vi "Handle TS Panel Results.vi"(6 "Method":T1, 8 "error in":errorcluster, 11 "HTS Test Stand in":refnum<class "HTS Test Stand.lvclass">) -> (0 "error out":errorcluster, 3 "HTS Test Stand out":refnum<class "HTS Test Stand.lvclass">)   [LabVIEW 2019, in "Test Stands.lvlib" / "HTS Test Stand.lvclass"]
uses:
  HTS Test Stand.lvclass
  Results/Results Method.ctl
  Results/Results.lvlib
  Generic Test Stand/Generic Test Stand.lvclass
  C:/Users/wg/Documents/LV_Projects/test-stand/App/Generic Test Stand/Generic Test Stand.lvclass
  Results/HTS Results/HTS Results.lvclass
  Generic Test Stand/TS Panel Method.ctl
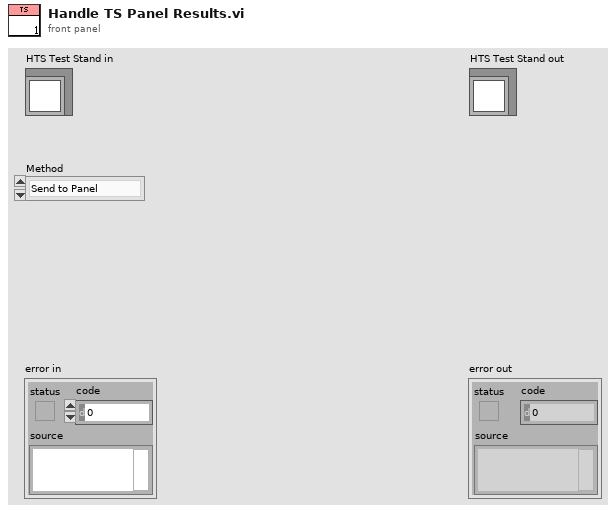
[diagram p1: front panel]
types:
  T1 = typedef "Generic Test Stand.lvclass/TS Panel Method.ctl" = enum16{"Send to Panel", "Receive from Panel"}
  T2 = typedef "Results.lvlib/Results Method.ctl" = enum16{"Get", "Set"}
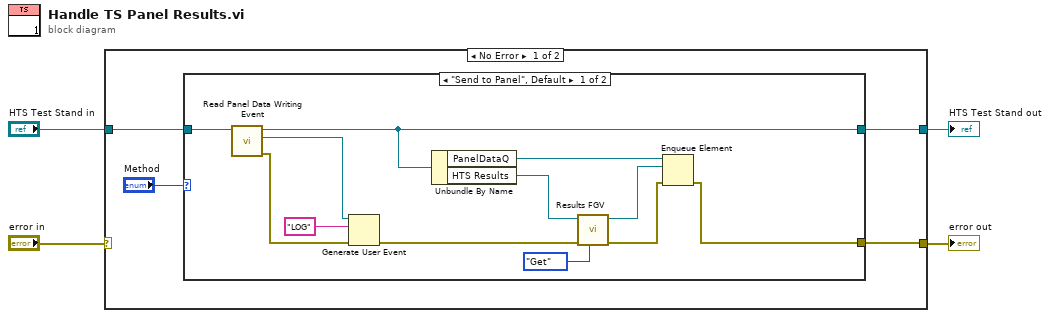
[diagram p0: block diagram]
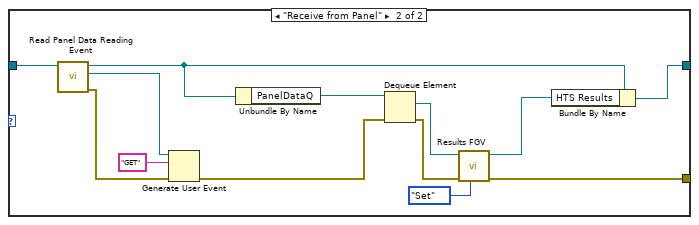
[diagram p2: hidden frame]
diagram:
  n1 = case shown="No Error" "error in" {
    selector: "error in" -> [_ w35]
    tunnel: [w7 w35] -> w2
    tunnel: [w6 w34] -> w1
    tunnel: "HTS Test Stand in" -> [w8 w34]
    frame No Error {
      n2 = case shown="\"Send to Panel\", Default" "Method" {
        tunnel: w8 -> [w13 w33]
        tunnel: [w11 w22] -> w7
        tunnel: [w12 w25] -> w6
        frame "Send to Panel", Default {
          n3 = call "Read Panel Data Writing Event.vi"("Generic Test Stand in"=w13) -> ("error out"=w10:errorcluster, "Panel Data Writing Event"=w14:refnum<user-event>, "Generic Test Stand out"=w12:refnum<class "HTS Test Stand.lvclass">)  [unwired: 8 in]
          n4 = Generate User Event(user event=w14, event data cluster="LOG" ("event data"), error in=w10) -> (error out=w16:errorcluster)  [unwired: 1 in, 1 out]
          n5 = Unbundle By Name(w12) -> ("PanelDataQ"=w18:refnum<queue>, "HTS Results"=w19:refnum<class "HTS Results.lvclass">)
          n6 = call-dynamic "Results FGV.vi"("Method"=Results_Method."Get", "error in"=w16, "HTS Results in"=w19) -> ("error out"=w15:errorcluster, "HTS Results out"=w17:refnum<class "HTS Results.lvclass">)  [unwired: 7 in]
          n7 = Enqueue Element(queue=w18, element=w17, error in (no error)=w15) -> (error out=w11:errorcluster)  [unwired: 1 in, 2 out]
        }
        frame "Receive from Panel" {
          n8 = call "Read Panel Data Reading Event.vi"("Generic Test Stand in"=w33) -> ("error out"=w30:errorcluster, "Panel Data Reading Event"=w32:refnum<user-event>, "Generic Test Stand out"=w28:refnum<class "HTS Test Stand.lvclass">)  [unwired: 8 in]
          n9 = Generate User Event(user event=w32, event data cluster="GET" ("event data"), error in=w30) -> (error out=w24:errorcluster)  [unwired: 1 in, 1 out]
          n10 = Unbundle By Name(w28) -> ("PanelDataQ"=w29:refnum<queue>)
          n11 = Dequeue Element(queue=w29, error in (no error)=w24) -> (element=w27:refnum<class "HTS Results.lvclass">, error out=w23:errorcluster)  [unwired: 1 in, 2 out]
          n12 = call-dynamic "Results FGV.vi"("Method"=Results_Method."Set", "error in"=w23, "HTS Results in"=w27) -> ("error out"=w22:errorcluster, "HTS Results out"=w26:refnum<class "HTS Results.lvclass">)  [unwired: 7 in]
          n13 = Bundle By Name(cluster=w28, "HTS Results"=w26) -> (w25:refnum<class "HTS Test Stand.lvclass">)
        }
      }
    }
    frame Error {
    }
  }
  "error out" <- w2
  "HTS Test Stand out" <- w1
